vi "Draw Flattened Pixmap (Fast)__jki_lib_picture -- VI Tester.vi"(8 "image data":T1, 9 "picture":picture) -> (3 "new picture":picture)   [LabVIEW 2011]
doc: "Draws a 1-, 4-, or 8-bit pixmap or a 24-bit RGB pixmap into a picture.\nThis VI is about 10% faster than NI original for 1 to 24-bit images without mask. For 32-bit images this is about 80% faster. For 1 to 24-bit images with mask, there is no differrence of speed."
uses:
  <vilib>/picture/picture.llb/imagedata.ctl
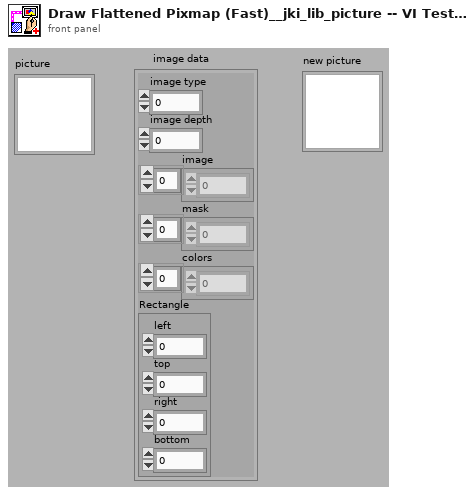
[diagram p1: front panel]
types:
  T1 = typedef "imagedata.ctl" = cluster{"image type":i32, "image depth":i32, "image":u8[], "mask":u8[], "colors":u32[], "Rectangle":cluster{"left":i16, "top":i16, "right":i16, "bottom":i16}}
  T2 = cluster{"left":i16, "top":i16, "right":i16, "bottom":i16}
  T3 = cluster{"top":i16, "left":i16, "bottom":i16, "right":i16}
  T4 = cluster{"default foreground":u32, "default background":u32}
  T5 = cluster{"opcode-Copy Pixmap":i16, i32, i32, cluster{"top":i16, "left":i16, "bottom":i16, "right":i16}, i16, cluster{"default foreground":u32, "default background":u32}}
  T6 = cluster{"opcode-Copy Pixmap w/Mask":i16, i32, i32, cluster{"top":i16, "left":i16, "bottom":i16, "right":i16}, i16, cluster{"default foreground":u32, "default background":u32}}
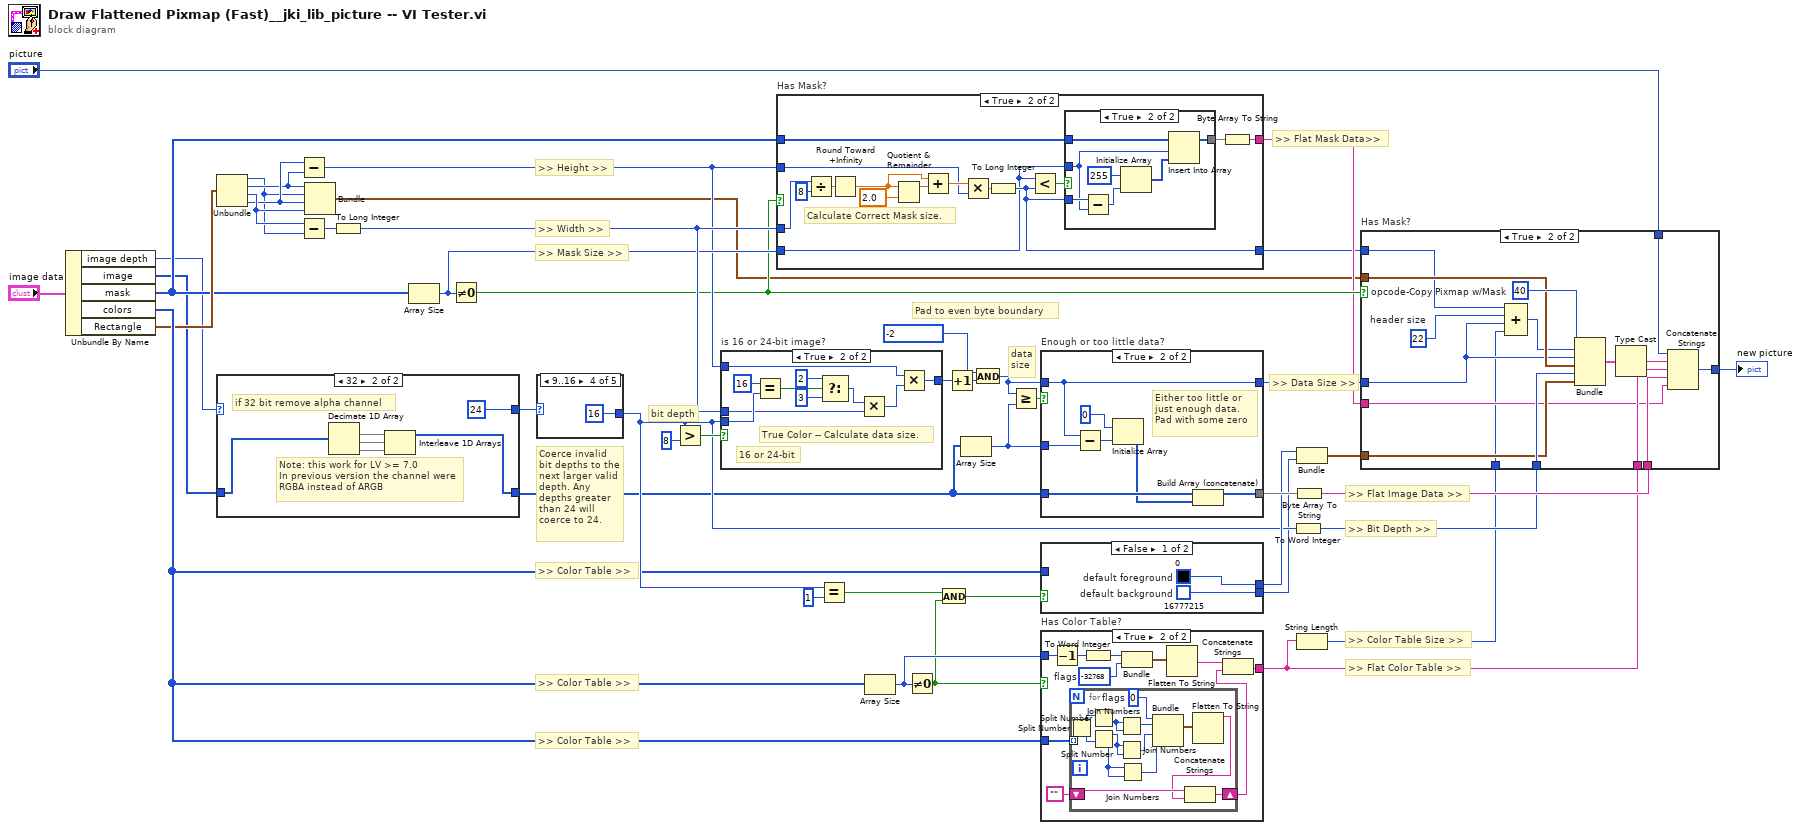
[diagram p0: block diagram]
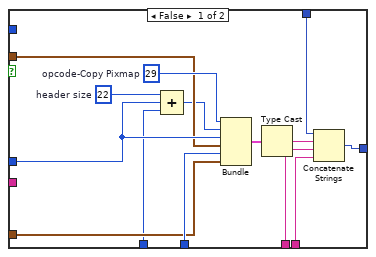
[diagram p2: hidden frame]
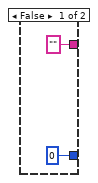
[diagram p3: hidden frame]
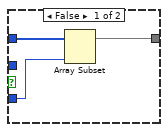
[diagram p4: hidden frame]
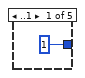
[diagram p6: hidden frame]
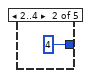
[diagram p7: hidden frame]
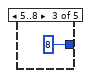
[diagram p8: hidden frame]
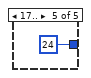
[diagram p9: hidden frame]
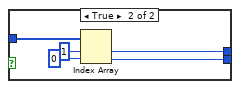
[diagram p10: hidden frame]
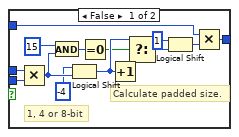
[diagram p11: hidden frame]
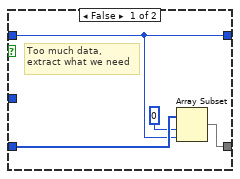
[diagram p12: hidden frame]
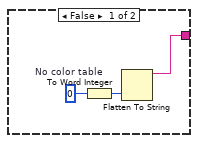
[diagram p13: hidden frame]
diagram:
  # ">> Mask Size >>"
  # ">> Flat Mask Data>>"
  # ">> Data Size >>"
  # ">> Flat Image Data >>"
  # ">> Flat Color Table >>"
  # ">> Color Table Size >>"
  # ">> Bit Depth >>"
  # "data\nsize"
  # ">> Height >>"
  # ">> Width >>"
  # ">> Color Table >>"
  # ">> Color Table >>"
  # ">> Color Table >>"
  # "Pad to even byte boundary"
  # "Coerce invalid bit depths to the next larger valid depth. Any depths greater than 24 will coerce to 24."
  # "bit depth"
  n1 = Unbundle By Name("image data") -> ("image depth"=w22:i32, "image"=w21:u8[], "mask"=w25:u8[], "colors"=w27:u32[], "Rectangle"=w26:T2)
  n2 = Unbundle(w26) -> ("left"=w24:i16, "top"=w42:i16, "right"=w44:i16, "bottom"=w43:i16)
  n3 = case shown="32" w22 {
    selector: w22 -> [w47 _]
    tunnel: [w47 24] -> w19
    tunnel: w21 -> [w46 w51]
    tunnel: [w46 w52] -> w20
    frame 1, 2, 4, 8, 24, Default {
    }
    frame 32 {
      # "Note: this work for LV >= 7.0\nIn previous version the channel were RGBA instead of ARGB"
      # "if 32 bit remove alpha channel"
      n4 = Decimate 1D Array(w51) -> (w49:u8[], w50:u8[], w48:u8[])  [unwired: 1 out]
      n5 = Interleave 1D Arrays(w49, w50, w48) -> (w52:u8[])
    }
  }
  n6 = Subtract(x=w43, y=w42) -> (x-y=w13:i16)
  n7 = Subtract(x=w44, y=w24) -> (x-y=w29:i16)
  n8 = Bundle("top"=w42, "left"=w24, "bottom"=w43, "right"=w44) -> (w5:T3)  [unwired: 1 in]
  n9 = To Long Integer(number=w29) -> (32bit integer=w23:i32)
  n10 = Array Size(array=w25) -> (size(s)=w14:i32)
  n11 = Not Equal To 0?(x=w14) -> (x != 0?=w12:bool)
  n12 = case shown="9..16" w19 {
    tunnel: [1 4 8 16 24] -> w31
    frame ..1 {
    }
    frame 2..4 {
    }
    frame 5..8 {
    }
    frame 9..16 {
    }
    frame 17.. {
    }
  }
  n13 = Greater?(x=w31, y=u8 8) -> (0:w37:bool)
  n14 = case "is 16 or 24-bit image?" shown="True" w37 {
    tunnel: [w72 w82] -> w16
    tunnel: w13 -> [w68 w81]
    tunnel: w31 -> [w60 w79]
    tunnel: w23 -> [w59 w77]
    frame False {
      # "1, 4 or 8-bit"
      # "Calculate padded size."
      n15 = Multiply(x=w59, y=w60) -> (x*y=w62:i32)
      n16 = And(x=15, y=w62) -> (x .and. y?=w64:i32)
      n17 = Logical Shift(y=-4, x=w62) -> (x << y=w66:i32)
      n18 = Equal To 0?(x=w64) -> (x = 0?=w65:bool)
      n19 = Increment(x=w66) -> (x+1=w67:i32)
      n20 = Select(t=w66, s=w65, f=w67) -> (s? t:f=w70:i32)
      n21 = Logical Shift(y=1, x=w70) -> (x << y=w71:i32)
      n22 = Multiply(x=w68, y=w71) -> (x*y=w72:i32)
    }
    frame True {
      # "16 or 24-bit"
      # "True Color -- Calculate data size."
      n23 = Equal?(x=16, y=w79) -> (x = y?=w76:bool)
      n24 = Select(t=2, s=w76, f=3) -> (s? t:f=w73:i32)
      n25 = Multiply(x=w73, y=w77) -> (x*y=w80:i32)
      n26 = Multiply(x=w81, y=w80) -> (x*y=w82:i32)
    }
  }
  n27 = case "Has Mask?" shown="True" w12 {
    tunnel: [0 w91] -> w8
    tunnel: w25 -> [_ w90]
    tunnel: ["" w88] -> w10
    tunnel: w23 -> [_ w87]
    tunnel: w14 -> [_ w86]
    tunnel: w13 -> [_ w85]
    frame False {
    }
    frame True {
      # "Calculate Correct Mask size."
      n28 = Divide(x=w87, y=8) -> (x/y=w96:dbl)
      n29 = Round Toward +Infinity(x=w96) -> (ceil(x): smallest int >= x=w95:dbl)
      n30 = Quotient & Remainder(x=w95, y=2.0) -> (x-y*floor(x/y)=w98:dbl)  [unwired: 1 out]
      n31 = Add(x=w95, y=w98) -> (x+y=w93:dbl)
      n32 = Multiply(x=w93, y=w85) -> (x*y=w97:dbl)
      n33 = To Long Integer(number=w97) -> (32bit integer=w91:i32)
      n34 = Less?(x=w86, y=w91) -> (x < y?=w92:bool)
      n35 = case shown="True" w92 {
        tunnel: w90 -> [w102 w105]
        tunnel: w86 -> [_ w104]
        tunnel: w91 -> [w101 w108]
        tunnel: [w100 w103] -> w89
        frame False {
          n36 = Array Subset(array=w102, length=w101) -> (w100:u8[])  [unwired: 1 in]
        }
        frame True {
          n37 = Subtract(x=w108, y=w104) -> (x-y=w107:i32)
          n38 = Initialize Array(u8 255 ("element"), w107) -> (w106:u8[])
          n39 = Insert Into Array(array=w105, index=w104, new element=w106) -> (w103:u8[])
        }
      }
      n40 = Byte Array To String(unsigned byte array=w89) -> (string=w88:string)
    }
  }
  n41 = Equal?(x=w31, y=u8 1) -> (x = y?=w32:bool)
  n42 = Array Size(array=w27) -> (size(s)=w45:i32)
  n43 = Not Equal To 0?(x=w45) -> (x != 0?=w34:bool)
  n44 = And(x=w32, y=w34) -> (x .and. y?=w35:bool)
  n45 = Increment(x=w16) -> (x+1=w18:i32)
  n46 = Array Size(array=w20) -> (size(s)=w40:i32)
  n47 = And(x=-2, y=w18) -> (x .and. y?=w15:i32)
  n48 = Greater Or Equal?(x=w15, y=w40) -> (x >= y?=w41:bool)
  n49 = case "Enough or too little data?" shown="True" w41 {
    tunnel: w20 -> [w113 w117]
    tunnel: [w112 w118] -> w39
    tunnel: w15 -> [w110 w114]
    tunnel: [w110 w114] -> w9
    tunnel: w40 -> [_ w115]
    frame False {
      # "Too much data, extract what we need"
      n50 = Array Subset(array=w113, index=0, length=w110) -> (w112:u8[])
    }
    frame True {
      # "Either too little or\njust enough data.\nPad with some zero"
      n51 = Subtract(x=w114, y=w115) -> (x-y=w120:i32)
      n52 = Initialize Array(u8 0, w120) -> (w116:u8[])
      n53 = Build Array (concatenate)(w117, w116) -> (w118:u8[])
    }
  }
  n54 = case shown="False" w35 {
    tunnel: [w122 w125] -> w36
    tunnel: [w121 w123] -> w30
    tunnel: w27 -> [_ w126]
    frame False {
      w121 = u32 16777215  # default background
      w122 = u32 0  # default foreground
    }
    frame True {
      n55 = Index Array(array=w126, index #1=1, index #2=0 ("index")) -> (element #1=w125:u32, element #2=w123:u32)
    }
  }
  n56 = case "Has Color Table?" shown="True" w34 {
    tunnel: w27 -> [_ w131]
    tunnel: w45 -> [_ w140]
    tunnel: [w128 w135] -> w3
    frame False {
      w130 = 0  # No color table
      n57 = To Word Integer(number=w130) -> (16bit integer=w129:i16)
      n58 = Flatten To String(anything=w129) -> (data string=w128:string)  [unwired: 3 in, 2 out]
    }
    frame True {
      w138 = i16 -32768  # flags
      n59 = Decrement(x=w140) -> (x-1=w132:i32)
      n60 = for {
        tunnel: w131 -> [w152] mode=indexing
        shift-right: [w149] -> w133
        shift-left: "" -> [w150]
        w151 = i16 0  # flags
        n61 = Split Number(x=w152) -> (hi(x)=w154:u16, lo(x)=w153:u16)
        n62 = Split Number(x=w154) -> (lo(x)=w141:u8)  [unwired: 1 out]
        n63 = Split Number(x=w153) -> (hi(x)=w147:u8, lo(x)=w146:u8)
        n64 = Join Numbers(hi=w141, lo=w141) -> ((hi.lo)=w148:u16)
        n65 = Join Numbers(hi=w147, lo=w147) -> ((hi.lo)=w145:u16)
        n66 = Join Numbers(hi=w146, lo=w146) -> ((hi.lo)=w144:u16)
        n67 = Bundle("flags"=w151, w148, w145, w144) -> (w143:cluster{"flags":i16, u16, u16, u16})  [unwired: 1 in]
        n68 = Flatten To String(anything=w143) -> (data string=w142:string)  [unwired: 3 in, 2 out]
        n69 = Concatenate Strings(w150, w142) -> (w149:string)
      }
      n70 = To Word Integer(number=w132) -> (16bit integer=w139:i16)
      n71 = Bundle(w139, "flags"=w138) -> (w137:cluster{i16, "flags":i16})  [unwired: 1 in]
      n72 = Flatten To String(anything=w137) -> (data string=w136:string)  [unwired: 3 in, 2 out]
      n73 = Concatenate Strings(w136, w133) -> (w135:string)
    }
  }
  n74 = To Word Integer(number=w31) -> (16bit integer=w2:i16)
  n75 = Byte Array To String(unsigned byte array=w39) -> (string=w4:string)
  n76 = Bundle("default foreground"=w36, "default background"=w30) -> (w11:T4)  [unwired: 1 in]
  n77 = String Length(string=w3) -> (length=w1:i32)
  n78 = case "Has Mask?" shown="True" w12 {
    tunnel: w1 -> [w156 w170]
    tunnel: w2 -> [w161 w182]
    tunnel: [w157 w181] -> w6
    tunnel: w3 -> [w163 w180]
    tunnel: w4 -> [w162 w179]
    tunnel: w11 -> [w160 w177]
    tunnel: w5 -> [w159 w176]
    tunnel: w9 -> [w164 w171]
    tunnel: w8 -> [_ w175]
    tunnel: w10 -> [_ w172]
    tunnel: "picture" -> [w158 w173]
    frame False {
      w167 = i16 22  # header size
      w165 = i16 29  # opcode-Copy Pixmap
      n79 = Compound Arithmetic op=ADD(w167, w164, w156) -> (w155:i32)
      n80 = Bundle("opcode-Copy Pixmap"=w165, w155, w164, w159, w161, w160) -> (w166:T5)  [unwired: 1 in]
      n81 = Type Cast(x=w166) -> (*(type *) &x=w168:string)  [unwired: 1 in]
      n82 = Concatenate Strings(w158, w168, w163, w162) -> (w157:picture)
    }
    frame True {
      w184 = i16 40  # opcode-Copy Pixmap w/Mask
      w174 = i16 22  # header size
      n83 = Compound Arithmetic op=ADD(w175, w174, w171, w170) -> (w169:i32)
      n84 = Bundle("opcode-Copy Pixmap w/Mask"=w184, w169, w171, w176, w182, w177) -> (w183:T6)  [unwired: 1 in]
      n85 = Type Cast(x=w183) -> (*(type *) &x=w178:string)  [unwired: 1 in]
      n86 = Concatenate Strings(w173, w178, w180, w179, w172) -> (w181:picture)
    }
  }
  "new picture" <- w6
